vi "Test Case, Array Limit Check.vi"() -> ()   [LabVIEW 2010]
panel:
  in  "lower fill":dbl=0.01 format="%.2f"
  in  "upper fill":dbl=0.25 format="%.2f"
  out "lower limit (delete)":dbl[][](array[numeric]) format="%.2f"
  in  "lower limit":dbl=0.25 format="%.2f"
  in  "upper limit":dbl=3.0 format="%.2f"
  out "pass count":dbl=nan
  in  "results":dbl[][](array[numeric])=[[1.5, 0.5], [2.5, 5.0], [0.0, 2.0]] format="%.2f"
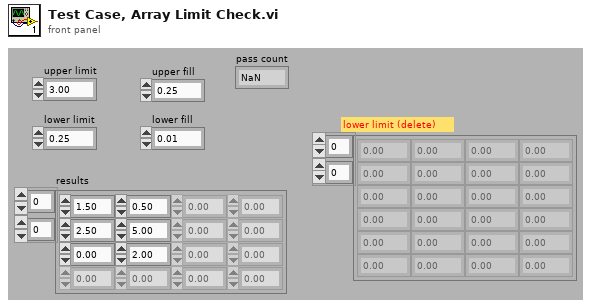
[diagram p1: front panel]
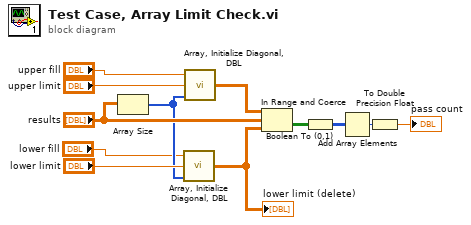
[diagram p0: block diagram]
diagram:
  n1 = Array Size(array="results") -> (size(s)=w6:i32[])
  n2 = call "Array, Initialize Diagonal, DBL.vi"("dimension"=w6, "diagonal"="lower limit", "fill"="lower fill") -> ("new array"=w7:dbl[][])
  "lower limit (delete)" <- w7
  n3 = call "Array, Initialize Diagonal, DBL.vi"("dimension"=w6, "diagonal"="upper limit", "fill"="upper fill") -> ("new array"=w4:dbl[][])
  n4 = In Range and Coerce(upper limit=w4, x="results", lower limit=w7) -> (In Range?=w12:bool[][])  [unwired: 1 out]
  n5 = Boolean To (0,1)(Boolean=w12) -> (0, 1=w11:i16[][])
  n6 = Add Array Elements(numeric array=w11) -> (sum=w10:i16)
  n7 = To Double Precision Float(number=w10) -> (double precision float=→"pass count":dbl)
